vi "Get state vector.vi"(8 "error in (no error)":errorcluster, 11 "G-UE in":refnum<class "G-UE.lvclass">) -> (0 "error out":errorcluster, 2 "State vector":cdb[](array[numeric]) format="%#_3g", 3 "G-UE out":refnum<class "G-UE.lvclass">)   [LabVIEW 2016, in "G-UE.lvclass"]
uses:
  G-UE.lvclass
  G-UE.lvclass/G-UE.ctl
  <vilib>/Analysis/baseanly.llb/Complex A x Vector.vi
  <vilib>/Analysis/NI_AALBase.lvlib
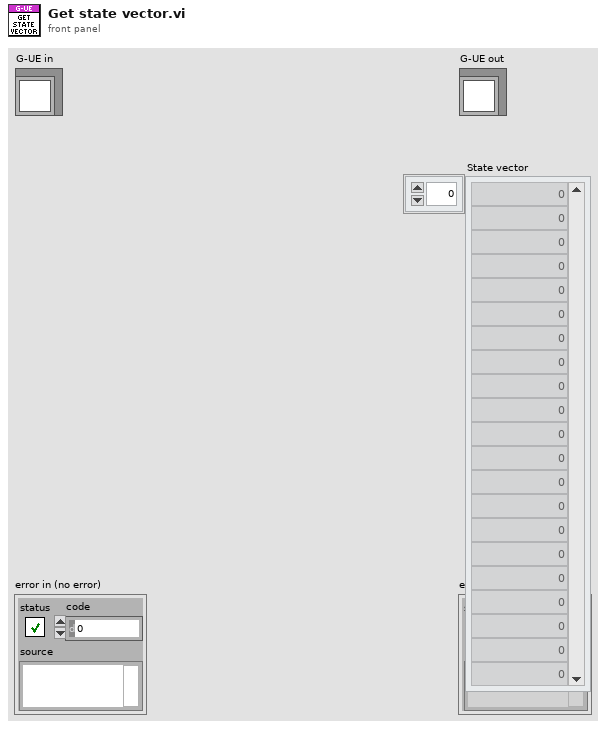
[diagram p1: front panel]
types:
  T1 = typedef "NI_Matrix.lvlib/ComplexMatrix.ctl" = cdb[][]
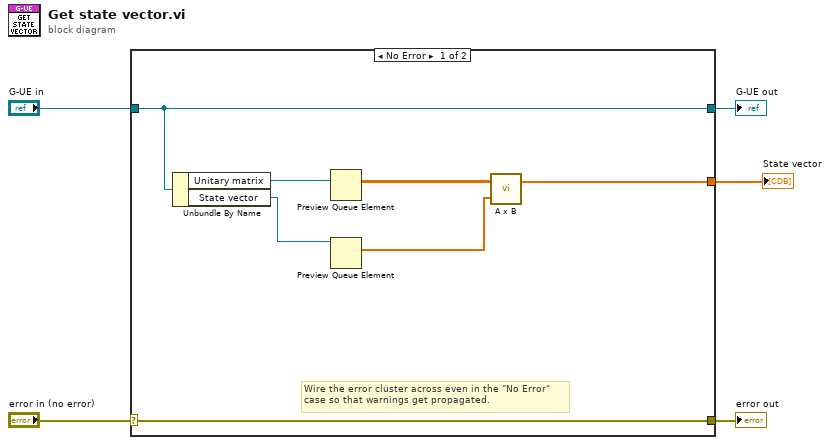
[diagram p0: block diagram]
diagram:
  n1 = case shown="No Error" "error in (no error)" {
    selector: "error in (no error)" -> [w12 w14]
    tunnel: [w12 w14] -> w4
    tunnel: [w10 w13] -> w2
    tunnel: "G-UE in" -> [w10 w13]
    tunnel: [w6 _] -> w1
    frame No Error {
      # "Wire the error cluster across even in the \"No Error\"\ncase so that warnings get propagated."
      n2 = Unbundle By Name(w10) -> ("Unitary matrix"=w9:refnum<queue>, "State vector"=w8:refnum<queue>)
      n3 = Preview Queue Element(queue=w9) -> (element=w11:T1)  [unwired: 2 in, 3 out]
      n4 = Preview Queue Element(queue=w8) -> (element=w7:cdb[])  [unwired: 2 in, 3 out]
      n5 = call-poly <vilib>:"A x B.vi"("Vector"=w7, "A"=w11) -> ("A x Vector"=w6:cdb[])  [unwired: 1 out]
    }
    frame Error {
    }
  }
  "error out" <- w4
  "G-UE out" <- w2
  "State vector" <- w1
